vi "Labview.vi"() -> ()   [LabVIEW 2010]
uses:
  <vilib>/Platform/TimedLoop/XDataNode/XDataNode.xnode
  <vilib>/Platform/TimedLoop/XDataNode/timing_clust.ctl
  <vilib>/Platform/TimedLoop/XDataNode/nitl_modes.ctl
  <vilib>/Platform/TimedLoop/XDataNode/wakeup.ctl
  <vilib>/Instr/_visa.llb/VISA Configure Serial Port (Instr).vi
  <vilib>/Platform/TimedLoop/XDataNode/XDNodeRunTimeDep.lvlib
panel:
  out "Numeric 2":i32
  out "Numeric":i32
  out "Manual":bool
  out "Auto":bool
  in  "Automatico/Manual":bool
  in  "Velocidad de Panel":u8(knob) scale=0.0..9.0
  out "Entrada sistema 2":dynamicdata(graph)
  in  "Period":i64=1000
  out "Puerto Serial":string
  in  "stop":bool
  in  "flow control":u16(ring) items=["None"=0, "XON/XOFF"=1, "RTS/CTS"=2, "DTR/DSR"=4]
  in  "stop bits":u16(ring)=10 items=["1.0"=10, "1.5"=15, "2.0"=20]
  in  "parity":u16(ring) items=["None", "Odd", "Even", "Mark", "Space"]
  in  "data bits":u16=8 min=5 max=8 step=1
  in  "VISA resource name":refnum<visa-resource-name>="COM1"
  in  "baud rate":u32=9600
  # "Proyecto de Instrumentación Industrial\n                                 Ing.Erwin Alejandro Moreira Alarcón                                      \n                                               PANEL SOLAR"
  # "COM SERIAL"
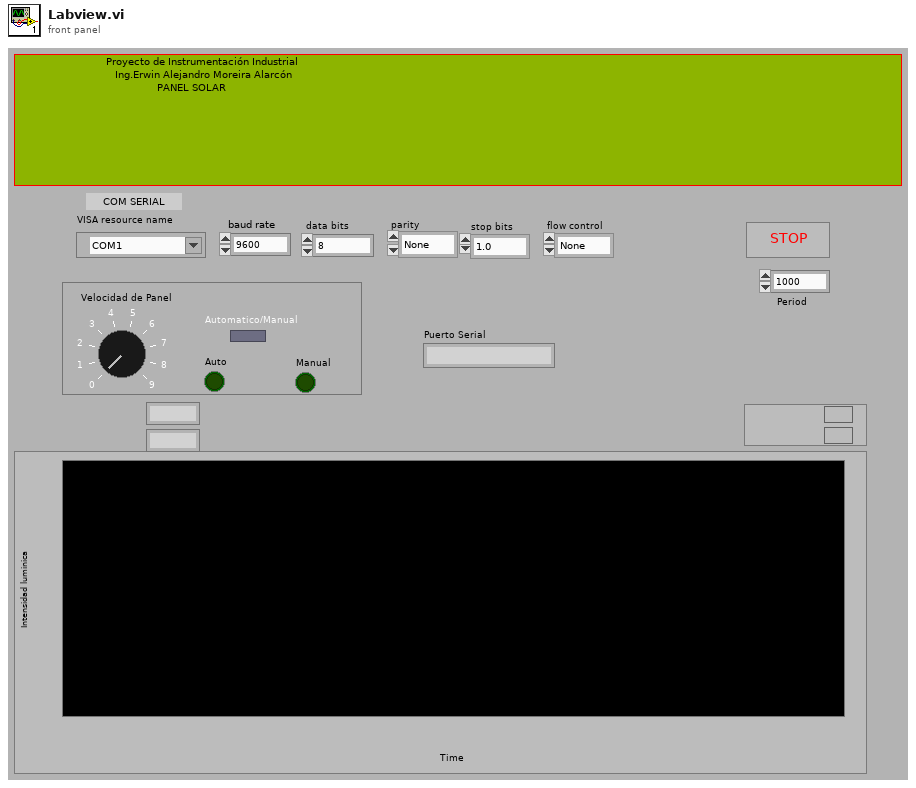
[diagram p1: front panel]
types:
  T1 = typedef "XDNodeRunTimeDep.lvlib/timing_clust.ctl" = cluster{"Expected End [f-1]":u64, "Actual End [f-1]":u64, "Finished Late? [f-1]":bool, "Expected End [i-1]":u64, "Actual End [i-1]":u64, "Finished Late? [i-1]":bool, "Expected Start [i]":u64, "Actual Start [i]":u64, "Expected Start [f]":u64, "Actual Start [f]":u64, "Source Name":string, "Structure Name":string, "Period":i64, "Deadline":i64, "Offset":i64, "Start":i64, "Priority":i32, "Timeout":i32, "Mode":T2, "Wakeup Reason":T3, "Error":errorcluster, "Source Type":string, "Secondary Source Type":string, "Global End Time":u64, "Global Start Time":u64, "Frame Duration":u64, "Iteration Duration":u64, "Assigned CPU":i32, "I/O Scan Engine Mode":u32}
  T2 = typedef "XDNodeRunTimeDep.lvlib/nitl_modes.ctl" = enum32{"No Change", "Process missed periods, maintain original phase", "Discard missed periods, maintain original phase", "Process missed periods, ignore original phase", "Discard missed periods, ignore original phase"}
  T3 = typedef "XDNodeRunTimeDep.lvlib/wakeup.ctl" = enum32{"Normal", "Aborted", "Asynchronous wakeup", "Timing source error", "Timed loop error", "Timeout"}
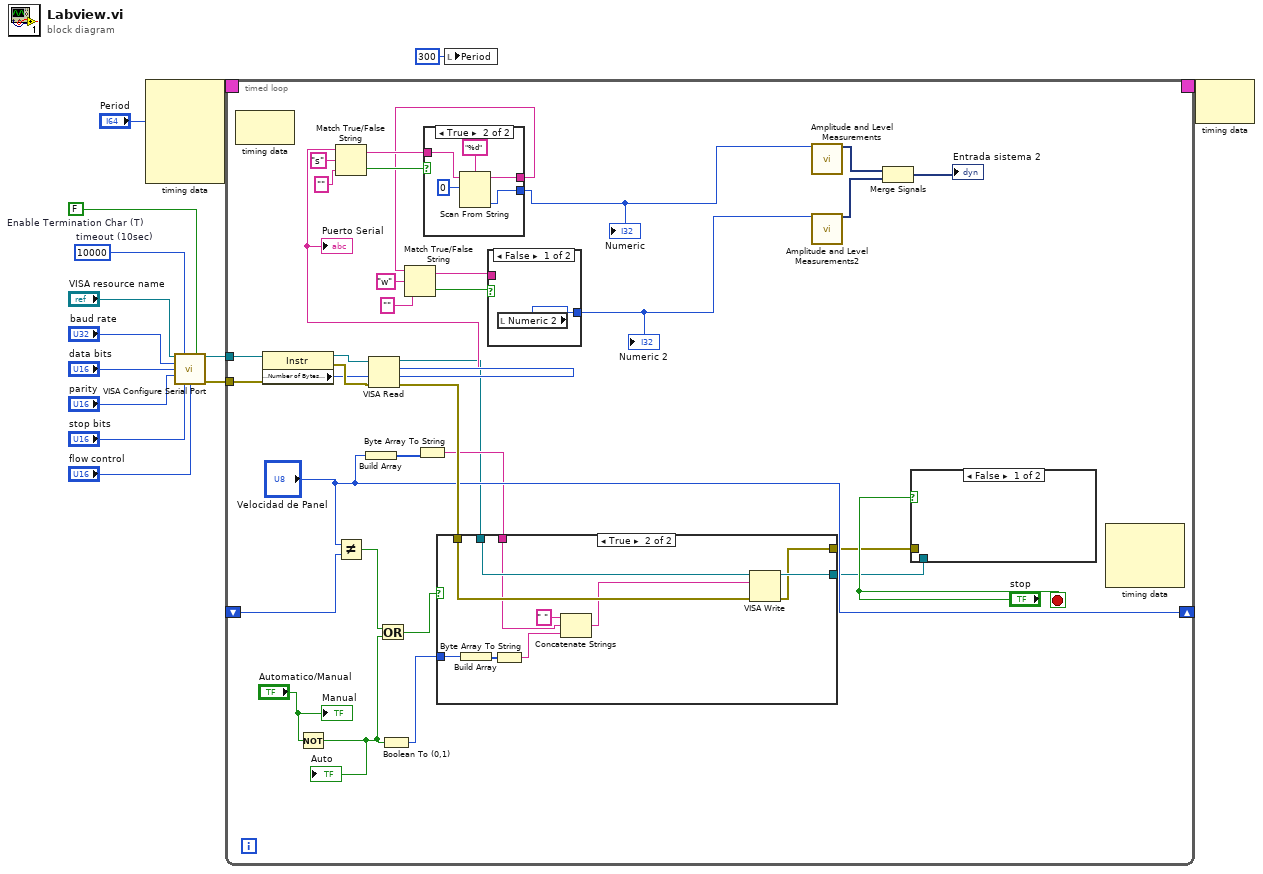
[diagram p0: block diagram]
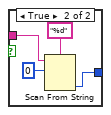
[diagram p3: hidden frame]
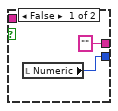
[diagram p4: hidden frame]
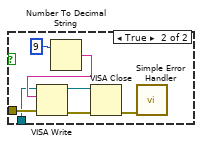
[diagram p5: hidden frame]
diagram:
  w8 = FALSE  # Enable Termination Char (T)
  w9 = u32 10000  # timeout (10sec)
  n1 = node-c288("Period") -> (w14:T1)  [unwired: 4 in]
  n2 = call-poly "VISA Configure Serial Port"("VISA resource name"="VISA resource name", "timeout (10sec)"=w9, "Enable Termination\nChar (T)"=w8, "baud rate (9600)"="baud rate", "data bits (8)"="data bits", "parity (0:none)"="parity", "stop bits (10: 1 bit)"="stop bits", "flow control (0:none)"="flow control") -> ("VISA resource name out"=w4:refnum<visa-resource-name>, "error out"=w3:errorcluster)  [unwired: 6 in]
  n3 = timed-loop {
    timing: w14 -> [_]
    timing-out: [_] -> w13
    tunnel: w4 -> [w32]
    tunnel: w3 -> [w31]
    shift-right: ["Velocidad de Panel"] -> _
    shift-left: _ -> [w29]
    stop <- "stop" stop-if-true
    n4 = node-c288() -> ()  [unwired: 1 in, 1 out]
    n5 = property class="Instr"(reference=w32, error in=w31) -> (reference out=w35:refnum<visa-resource-name>, error out=w48:errorcluster, "Serial Settings:Number of Bytes at Serial Port"=w47:u32)
    n6 = Not(x="Automatico/Manual") -> (.not. x?=w19:bool)
    "Auto" <- w19
    n7 = Not Equal?(x="Velocidad de Panel", y=w29) -> (x != y?=w20:bool)
    n8 = Build Array("Velocidad de Panel") -> (w26:u8[])
    n9 = VISA Read(VISA resource name=w35, byte count=w47, error in (no error)=w48) -> (VISA resource name out=w24:refnum<visa-resource-name>, read buffer=w45:string, error out=w28:errorcluster)  [unwired: 1 out]
    "Puerto Serial" <- w45
    n10 = Match True/False String(2:"" ("false string"), 3:"s" ("true string"), 4:w45) -> (0:w43:bool, 1:w42:string)
    n11 = Or(x=w20, y=w19) -> (x .or. y?=w17:bool)
    n12 = Boolean To (0,1)(Boolean=w19) -> (0, 1=w18:i16)
    n13 = Byte Array To String(unsigned byte array=w26) -> (string=w25:string)
    n14 = case shown="True" w43 {
      tunnel: w42 -> [_ w70]
      tunnel: ["" w69] -> w40
      tunnel: [w66 w68] -> w22
      frame False {
        n15 = local read "Numeric"() -> (w66:i32)
      }
      frame True {
        n16 = Scan From String(format string="%d", input string=w70, initial scan location=u32 0) -> (remaining string=w69:string, output 1=w68:i32)  [unwired: 2 in, 2 out]
      }
    }
    "Numeric" <- w22
    n17 = Match True/False String(2:"" ("false string"), 3:"w" ("true string"), 4:w40) -> (0:w38:bool, 1:w39:string)
    n18 = case shown="True" w17 {
      tunnel: w28 -> [w50 w59]
      tunnel: w25 -> [_ w57]
      tunnel: w24 -> [w49 w60]
      tunnel: w18 -> [_ w55]
      tunnel: [w49 w52] -> w15
      tunnel: [w50 w51] -> w16
      frame False {
      }
      frame True {
        n19 = Build Array(w55) -> (w54:i16[])
        n20 = Byte Array To String(unsigned byte array=w54) -> (string=w53:string)
        n21 = Concatenate Strings(" " ("string"), w57, w53) -> (w56:string)
        n22 = VISA Write(VISA resource name=w60, write buffer=w56, error in (no error)=w59) -> (VISA resource name out=w52:refnum<visa-resource-name>, error out=w51:errorcluster)  [unwired: 1 out]
      }
    }
    n23 = case shown="False" w38 {
      tunnel: w39 -> [_ w63]
      tunnel: [w61 w62] -> w21
      frame False {
        n24 = local read "Numeric 2"() -> (w61:i32)
      }
      frame True {
        n25 = Scan From String(format string="%d", input string=w63, initial scan location=u32 0) -> (output 1=w62:i32)  [unwired: 2 in, 3 out]
      }
    }
    "Numeric 2" <- w21
    n26 = call "Amplitude and Level Measurements"("Signals"=w22) -> ("Mean (DC)"=w34:dynamicdata)  [unwired: 13 in, 1 out]
    n27 = call "Amplitude and Level Measurements2"("Signals"=w21) -> ("Mean (DC)"=w30:dynamicdata)  [unwired: 13 in, 1 out]
    n28 = Merge Signals(w34, w30) -> (→"Entrada sistema 2":dynamicdata)
    n29 = case shown="False" "stop" {
      tunnel: w16 -> [_ w74]
      tunnel: w15 -> [_ w73]
      frame False {
      }
      frame True {
        n30 = Number To Decimal String(number=9) -> (decimal integer string=w75:string)  [unwired: 1 in]
        n31 = VISA Write(VISA resource name=w73, write buffer=w75, error in (no error)=w74) -> (VISA resource name out=w77:refnum<visa-resource-name>, error out=w76:errorcluster)  [unwired: 1 out]
        n32 = VISA Close(VISA resource name=w77, error in (no error)=w76) -> (error out=w79:errorcluster)
        n33 = call <vilib>:"Simple Error Handler.vi"("error in (no error)"=w79) -> ()  [unwired: 4 in, 5 out]
      }
    }
    n34 = node-c288() -> ()  [unwired: 3 in, 1 out]
    "Manual" <- "Automatico/Manual"
  }
  n35 = local write "Period"(i64 300 ("Period")) -> ()
  n36 = node-c288(w13) -> ()  [unwired: 1 out]
